vi "MultiOpto_1.4_Begin.vi"() -> (9 "NI DMM 3 option return":enum32{"Ampermeter button", "Ohmmeter button"}(ring), 11 "NI DMM 2 option return":enum32{"Ampermeter button", "Ohmmeter button"}(ring), 13 "NI DMM 1 option return":enum32{"Ampermeter button", "Ohmmeter button"}(ring), 15 "Stepper Motor Status":bool, 17 "Ophir 2 Status":bool, 18 "Текущий Образец №":string, 19 "Ophir 1 Status":bool, 20 "DC Power 1 Status":bool, 21 "DC Power 2 Status":bool, 22 "DC Power 3 Status":bool, 23 "DC Power 4 Status":bool, 24 "NI DMM 1 Status":bool, 25 "NI DMM 2 Status":bool, 26 "NI DMM 3 Status":bool, 27 "NI Scope Status":bool)   [LabVIEW 2018]
panel:
  in  "DC Power 4":bool
  in  "DC Power 3":bool
  in  "DC Power 1":bool
  in  "DC Power 2":bool
  in  "OK Button":bool
  in  "Stepper Motor":bool
  in  "NI DMM 3 option":enum32{"Ampermeter button", "Ohmmeter button"}(radio)
  in  "NI DMM 3":bool
  in  "NI DMM 2 option":enum32{"Ampermeter button", "Ohmmeter button"}(radio)
  in  "NI DMM 1 option":enum32{"Ampermeter button", "Ohmmeter button"}(radio)
  in  "Ophir 2":bool
  in  "NI DMM 2":bool
  out "Boolean 4":bool
  out "Boolean 3":bool
  in  "Ophir 1":bool
  in  "NI DMM 1":bool
  in  "NI Scope":bool
  in  "Образец №":string
  out "Boolean":bool
  out "Boolean 2":bool
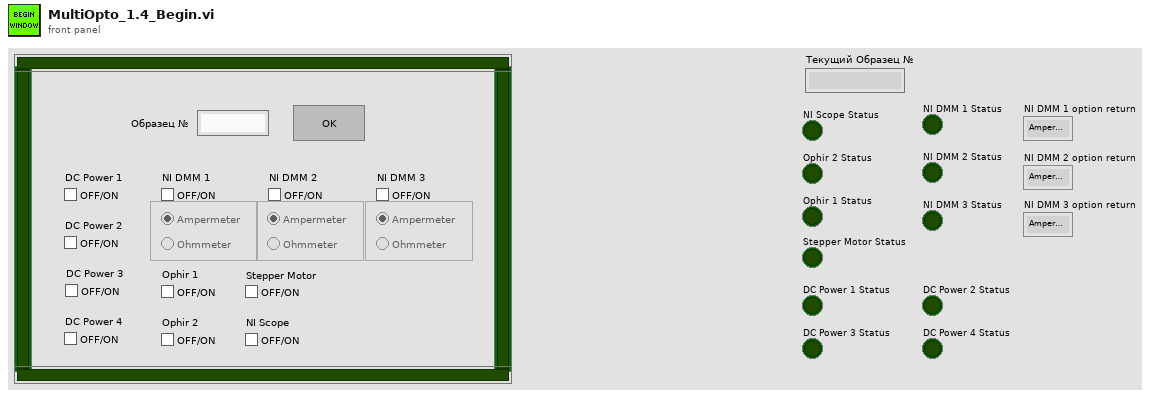
[diagram p1: front panel]
types:
  T1 = enum8{"Enabled", "Disabled", "Disabled and Grayed Out"}
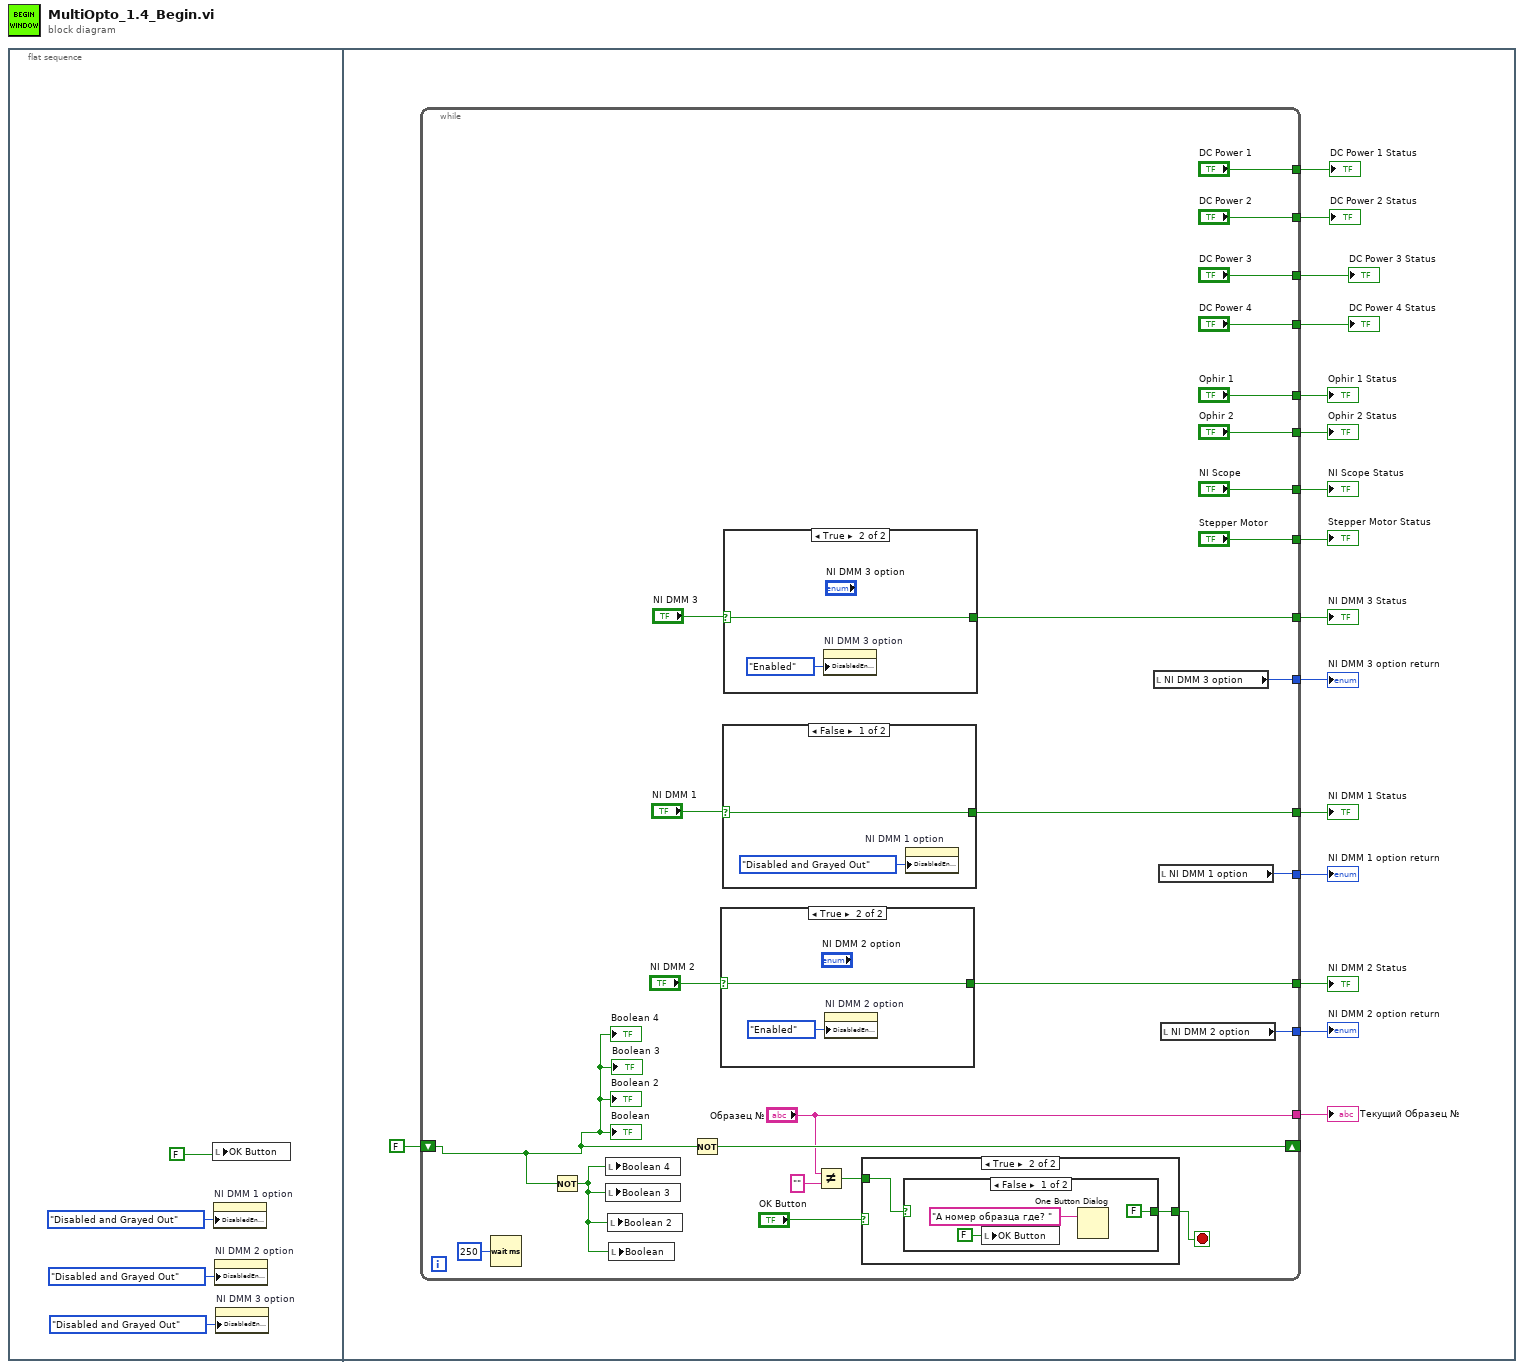
[diagram p0: block diagram]
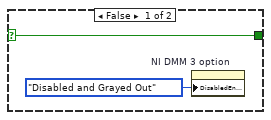
[diagram p4: hidden frame]
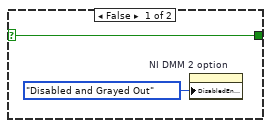
[diagram p5: hidden frame]
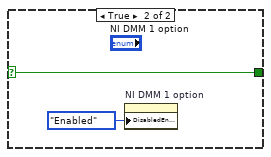
[diagram p6: hidden frame]
diagram:
  n1 = flat-sequence {
    frame #0 {
      n2 = local write "OK Button"(FALSE ("Ввел!")) -> ()
      n3 = property on="NI DMM 1 option" class="RadioBtnsControl (strict)"("DisabledEnum"=T1."Disabled and Grayed Out" ("Disabled")) -> ()  [unwired: 2 in, 2 out]
      n4 = property on="NI DMM 2 option" class="RadioBtnsControl (strict)"("DisabledEnum"=T1."Disabled and Grayed Out" ("Disabled")) -> ()  [unwired: 2 in, 2 out]
      n5 = property on="NI DMM 3 option" class="RadioBtnsControl (strict)"("DisabledEnum"=T1."Disabled and Grayed Out" ("Disabled")) -> ()  [unwired: 2 in, 2 out]
    }
    frame #1 {
      n6 = while {
        tunnel: ["Образец №"] -> w20
        shift-right: [w45] -> _
        shift-left: FALSE -> [w44]
        tunnel: ["NI Scope"] -> w18
        tunnel: [w37] -> w17
        tunnel: ["Ophir 1"] -> w16
        tunnel: [w36] -> w15
        tunnel: ["Ophir 2"] -> w14
        tunnel: [w35] -> w13
        tunnel: [w34] -> w12
        tunnel: [w32] -> w11
        tunnel: [w31] -> w10
        tunnel: ["Stepper Motor"] -> w9
        tunnel: ["DC Power 1"] -> w8
        tunnel: ["DC Power 2"] -> w7
        tunnel: ["DC Power 3"] -> w6
        tunnel: ["DC Power 4"] -> w5
        stop <- w27 stop-if-true
        n7 = Wait (ms)(milliseconds to wait=u32 250) -> ()  [unwired: 1 out]
        n8 = Not(x=w44) -> (.not. x?=w43:bool)
        n9 = local write "Boolean 4"(w43) -> ()
        n10 = local write "Boolean 3"(w43) -> ()
        n11 = local write "Boolean 2"(w43) -> ()
        n12 = local write "Boolean"(w43) -> ()
        n13 = Not(x=w44) -> (.not. x?=w45:bool)
        n14 = case shown="True" "NI DMM 2" {
          selector: "NI DMM 2" -> [w58 w61]
          tunnel: [w58 w61] -> w36
          frame False {
            n15 = property on="NI DMM 2 option" class="RadioBtnsControl (strict)"("DisabledEnum"=T1."Disabled and Grayed Out" ("Disabled")) -> ()  [unwired: 2 in, 2 out]
          }
          frame True {
            n16 = property on="NI DMM 2 option" class="RadioBtnsControl (strict)"("DisabledEnum"=T1."Enabled" ("Disabled")) -> ()  [unwired: 2 in, 2 out]
          }
        }
        n17 = case shown="False" "NI DMM 1" {
          selector: "NI DMM 1" -> [w62 w65]
          tunnel: [w62 w65] -> w37
          frame False {
            n18 = property on="NI DMM 1 option" class="RadioBtnsControl (strict)"("DisabledEnum"=T1."Disabled and Grayed Out" ("Disabled")) -> ()  [unwired: 2 in, 2 out]
          }
          frame True {
            n19 = property on="NI DMM 1 option" class="RadioBtnsControl (strict)"("DisabledEnum"=T1."Enabled" ("Disabled")) -> ()  [unwired: 2 in, 2 out]
          }
        }
        n20 = case shown="True" "NI DMM 3" {
          selector: "NI DMM 3" -> [w54 w57]
          tunnel: [w54 w57] -> w32
          frame False {
            n21 = property on="NI DMM 3 option" class="RadioBtnsControl (strict)"("DisabledEnum"=T1."Disabled and Grayed Out" ("Disabled")) -> ()  [unwired: 2 in, 2 out]
          }
          frame True {
            n22 = property on="NI DMM 3 option" class="RadioBtnsControl (strict)"("DisabledEnum"=T1."Enabled" ("Disabled")) -> ()  [unwired: 2 in, 2 out]
          }
        }
        n23 = Not Equal?(x="Образец №", y="") -> (x != y?=w28:bool)
        n24 = case shown="True" "OK Button" {
          selector: "OK Button" -> [w47 _]
          tunnel: w28 -> [_ w49]
          tunnel: [w47 w48] -> w27
          frame False {
          }
          frame True {
            n25 = case shown="False" w49 {
              selector: w49 -> [_ w53]
              tunnel: [FALSE w53] -> w48
              frame False {
                n26 = local write "OK Button"(FALSE ("OK Button")) -> ()
                n27 = One Button Dialog(message="А номер образца где? ") -> ()  [unwired: 1 in, 1 out]
              }
              frame True {
              }
            }
          }
        }
        n28 = local read "NI DMM 3 option"() -> (w31:enum32{"Ampermeter button", "Ohmmeter button"})
        n29 = local read "NI DMM 1 option"() -> (w35:enum32{"Ampermeter button", "Ohmmeter button"})
        n30 = local read "NI DMM 2 option"() -> (w34:enum32{"Ampermeter button", "Ohmmeter button"})
        "Boolean" <- w44
        "Boolean 2" <- w44
        "Boolean 3" <- w44
        "Boolean 4" <- w44
      }
      "Текущий Образец №" <- w20
      "NI Scope Status" <- w18
      "NI DMM 1 Status" <- w17
      "Ophir 1 Status" <- w16
      "NI DMM 2 Status" <- w15
      "Ophir 2 Status" <- w14
      "NI DMM 2 option return" <- w12
      "NI DMM 1 option return" <- w13
      "NI DMM 3 Status" <- w11
      "NI DMM 3 option return" <- w10
      "Stepper Motor Status" <- w9
      "DC Power 1 Status" <- w8
      "DC Power 2 Status" <- w7
      "DC Power 3 Status" <- w6
      "DC Power 4 Status" <- w5
    }
  }
